vi "mxwScript_API_XMLTemplateName_CreateControlIndicators.vi"(6 "createIndicators?":bool=TRUE, 7 "uniquify?":bool, 8 "error in (no error)":errorcluster, 9 "createControls?":bool=TRUE, 10 "nodePattern":string, 11 "absolutePath":string) -> (0 "error out":errorcluster, 3 "encoded absolutePath":string)   [LabVIEW 2020]
doc: "Create controls and/or indicators on a node on the template after the node is dropped. The node is identified with the match pattern string <B>nodePattern</B>."
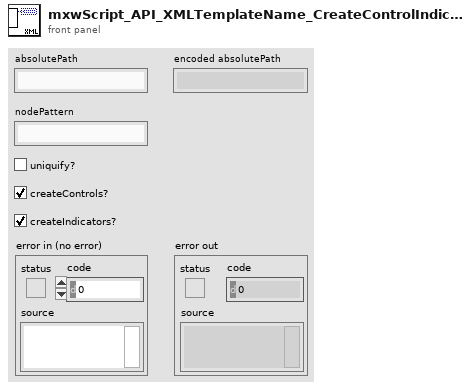
[diagram p1: front panel]
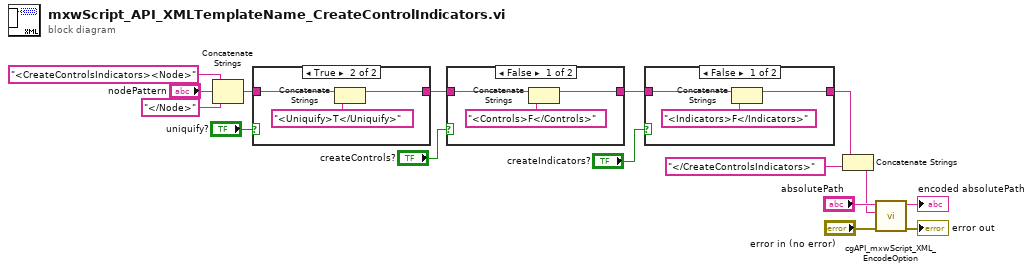
[diagram p0: block diagram]
diagram:
  n1 = Concatenate Strings("<CreateControlsIndicators><Node>" ("control name"), "nodePattern", "</Node>" ("string")) -> (w8:string)
  n2 = case shown="True" "uniquify?" {
    tunnel: w8 -> [w17 w20]
    tunnel: [w17 w18] -> w7
    frame False {
    }
    frame True {
      n3 = Concatenate Strings(w20, "<Uniquify>T</Uniquify>") -> (w18:string)
    }
  }
  n4 = case shown="False" "createControls?" {
    tunnel: w7 -> [w23 w24]
    tunnel: [w21 w24] -> w5
    frame False {
      n5 = Concatenate Strings(w23, "<Controls>F</Controls>") -> (w21:string)
    }
    frame True {
    }
  }
  n6 = case shown="False" "createIndicators?" {
    tunnel: w5 -> [w27 w28]
    tunnel: [w25 w28] -> w2
    frame False {
      n7 = Concatenate Strings(w27, "<Indicators>F</Indicators>") -> (w25:string)
    }
    frame True {
    }
  }
  n8 = Concatenate Strings(w2, "</CreateControlsIndicators>") -> (w1:string)
  n9 = call "cgAPI_mxwScript_XML_EncodeOption.vi"("error in (no error)"="error in (no error)", "otherXML"=w1, "normalTextString"="absolutePath") -> ("error out"=→"error out":errorcluster, "encodedString"=→"encoded absolutePath":string)  [unwired: 7 out]
